vi "Test Cases - float.vi"() -> ()   [LabVIEW 2017]
uses:
  4ee676fc-47c0-4be0-9ff8-88677d132e6f.vi
  a152669e-7808-472e-ac68-82058263c032.vi
  5d5e870e-b8ec-4111-8fcd-715cbb1e366c.vi
  6ca2ea0b-5a64-4cad-9736-18ec21bbeae0.vi
  API-String-Arugments-Support/_Support/Data To API String Arguments.vi
  API-String-Arugments-Support/_Support/Convert API String Arguments to Data(variant).vi
panel:
  out "Array 2":T1(array[cluster]) {"?" format="%#_6e"; "Data" format="%#_6e"}
  out "Array":T1(array[cluster]) {"?" format="%#_6e"; "Data" format="%#_6e"}
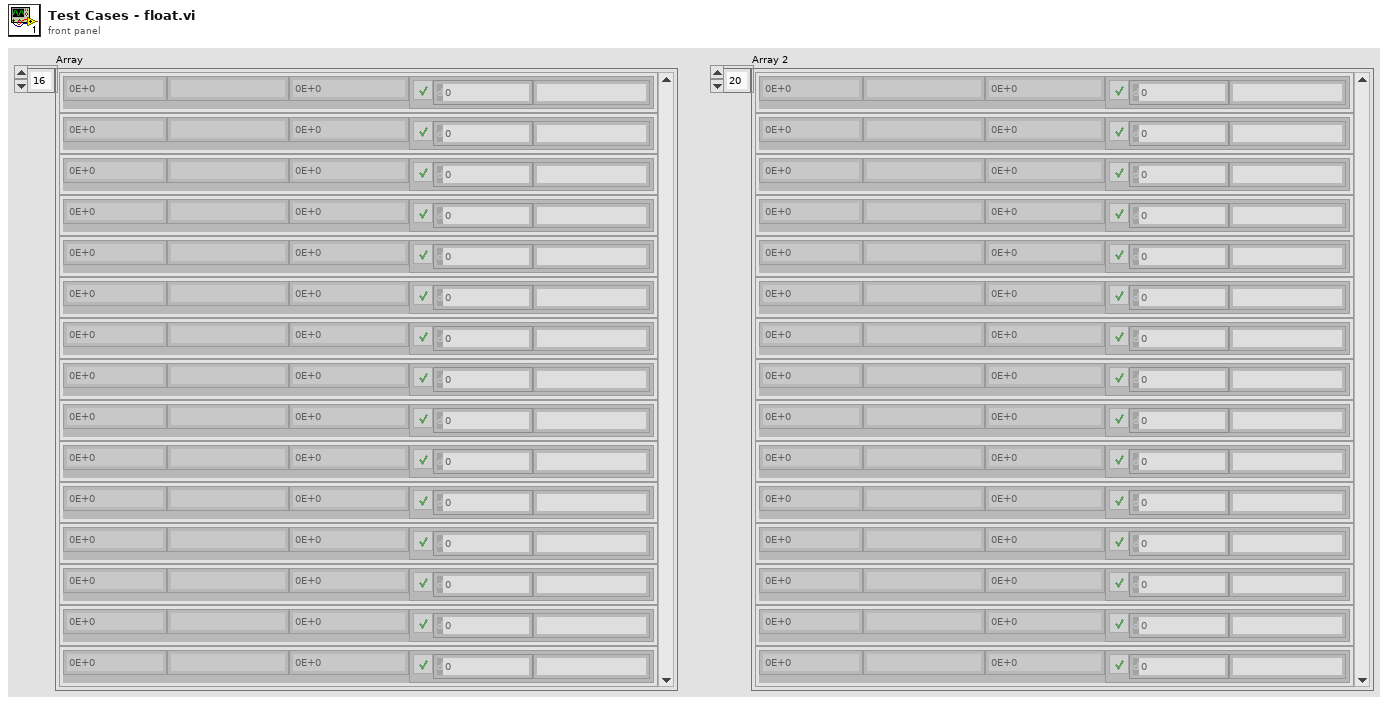
[diagram p1: front panel]
types:
  T1 = cluster{dbl, "String":string, "Data":dbl, "error":errorcluster}[]
  T2 = cluster{dbl, "String":string, "Data":dbl, "error":errorcluster}
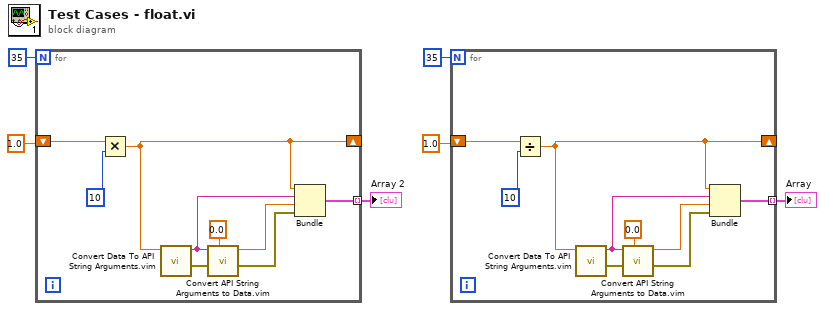
[diagram p0: block diagram]
diagram:
  n1 = for {
    N: 35 -> [_]
    shift-right: [w11] -> _
    shift-left: 1.0 -> [w14]
    tunnel: [w7] -> w3 mode=indexing
    n2 = Multiply(x=w14, y=10) -> (x*y=w11:dbl)
    n3 = call "Convert Data To API String Arguments.vim"("data"=w11) -> ("error out"=w12:errorcluster, "String"=w10:string)  [unwired: 7 in]
    n4 = call "Convert API String Arguments to Data.vim"("Type"=0.0, "error in (no error)"=w12, "String"=w10) -> ("error"=w8:errorcluster, "Data"=w9:dbl)  [unwired: 5 in]
    n5 = Bundle(w11, "String"=w10, "Data"=w9, "error"=w8) -> (w7:T2)  [unwired: 1 in]
  }
  "Array 2" <- w3
  n6 = for {
    N: 35 -> [_]
    shift-right: [w20] -> _
    shift-left: 1.0 -> [w23]
    tunnel: [w16] -> w4 mode=indexing
    n7 = Divide(x=w23, y=10) -> (x/y=w20:dbl)
    n8 = call "Convert Data To API String Arguments.vim"("data"=w20) -> ("error out"=w21:errorcluster, "String"=w19:string)  [unwired: 7 in]
    n9 = call "Convert API String Arguments to Data.vim"("Type"=0.0, "error in (no error)"=w21, "String"=w19) -> ("error"=w17:errorcluster, "Data"=w18:dbl)  [unwired: 5 in]
    n10 = Bundle(w20, "String"=w19, "Data"=w18, "error"=w17) -> (w16:T2)  [unwired: 1 in]
  }
  "Array" <- w4
